vi "UI_RunTest.vi"() -> ()   [LabVIEW 2017]
panel:
  in  "Data_Recorde":T1 caption="测试数据记录"
  in  "Speeds 2":i8 caption="环境温度" format="%1b"
  in  "Speeds":i8 caption="模拟运行速度" format="%1b"
  in  "Sum_Steps":i8 caption="运动总步数" format="%1b"
  in  "Shutdown":bool
  in  "Trouble Code":dbl caption="故障代码"
  out "Alarm":bool caption="故障报警"
  in  "Position_measure_data":T2 caption="棒位测量数据" {"Transfer_code" format="%1b"}
  in  "Orig_data":T3 caption="通道采样数据"
  out "Waveform Chart 2":dbl(graph)
  out "Waveform Chart":dbl(graph)
  in  "stop":bool
  out "T_time":string caption="试验时间"
  out "T_Date":string caption="试验日期"
  # "低温堆棒位测量试验系统"
  # "MB"
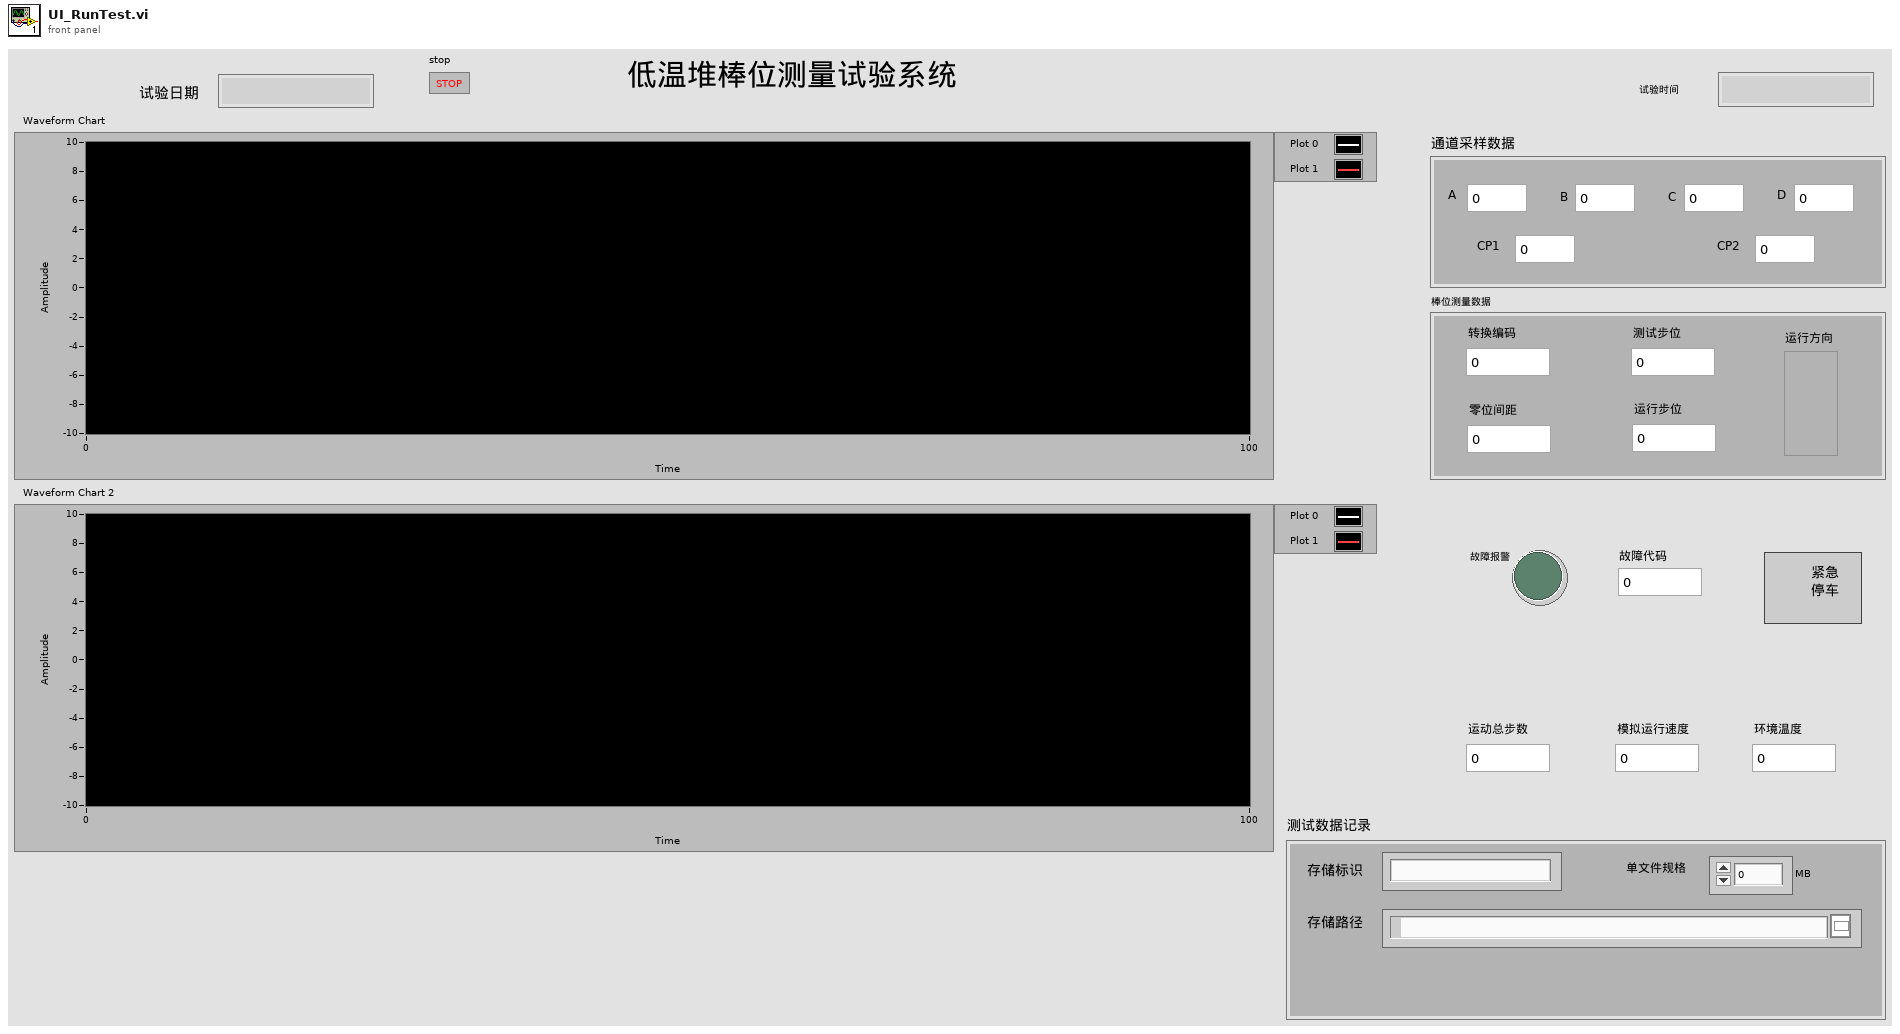
[diagram p1: front panel]
types:
  T1 = cluster{"Save_File_id":string, "File_Size":dbl, "File Path ":path}
  T2 = cluster{"Transfer_code":i8, "Test_Step":dbl, "Zero_Space":dbl, "Run_Step":dbl, "Direction":bool}
  T3 = cluster{"A":dbl, "B":dbl, "C":dbl, "D":dbl, "CP1":dbl, "CP2":dbl}
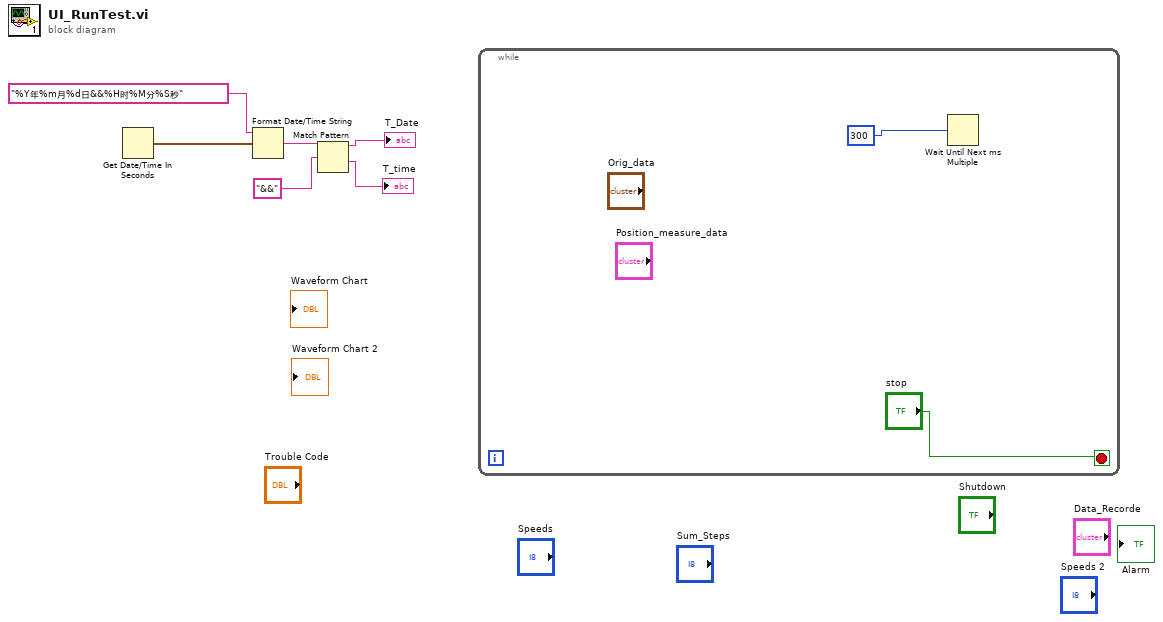
[diagram p0: block diagram]
diagram:
  n1 = Get Date/Time In Seconds() -> (seconds since 1Jan1904=w5:timestamp)
  n2 = Format Date/Time String(time format string (%c)="%Y年%m月%d日&&%H时%M分%S秒", seconds (now)=w5) -> (date/time string=w4:string)  [unwired: 1 in]
  n3 = Match Pattern(string=w4, regular expression="&&") -> (before substring=→"T_Date":string, after substring=→"T_time":string)  [unwired: 1 in, 2 out]
  n4 = while {
    stop <- "stop" stop-if-true
    n5 = Wait Until Next ms Multiple(millisecond multiple=300) -> ()  [unwired: 1 out]
  }
